vi "Control Path.vi"(11 "CheckboxControlEditorPanel in":refnum<class "CheckboxControlEditorPanel.lvclass">) -> (2 "Control Path":path[](array[path]))   [LabVIEW 2020, in "VolatusGUIControls.lvlib" / "CheckboxControlEditorPanel.lvclass"]
uses:
  CheckboxControlEditorPanel.lvclass
  CheckboxControlEditorPanel.lvclass/CheckboxControlEditorPanel.ctl
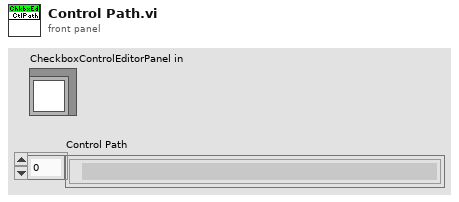
[diagram p1: front panel]
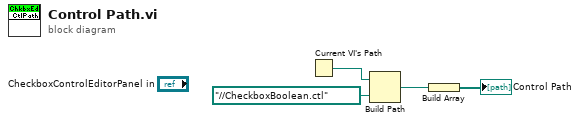
[diagram p0: block diagram]
diagram:
  n1 = Current VI's Path() -> (path=w4:path)
  n2 = Build Path(base path=w4, name or relative path=path "../../CheckboxBoolean.ctl") -> (appended path=w2:path)
  n3 = Build Array(w2) -> (→"Control Path":path[])
